vi "State_Machine.vi"(8 "error in (no error)":errorcluster caption="entrée d'erreur (pas d'erreur)", 11 "Generate_SN en entrée":refnum<class "Nodon_Generate_SN_Product.lvclass">) -> (0 "error out":errorcluster caption="sortie d'erreur", 2 "Json_String":string, 3 "Generate_SN en sortie":refnum<class "Nodon_Generate_SN_Product.lvclass">)   [LabVIEW 2020, in "Library Test.lvlib" / "Nodon_Generate_SN_Product.lvclass"]
uses:
  Nodon_Generate_SN_Product.lvclass
  C:/Users/ngarcin/OneDrive - Altyor/Standard TB/Class/Test/Find_SN_In_Database/Find_SN_In_Database.lvclass
  Find_SN_In_Database/Find_SN_In_Database.lvclass
  Nodon_Generate_SN_Product.lvclass/Nodon_Generate_SN_Product.ctl
  Commun VI/Library Commun.lvlib
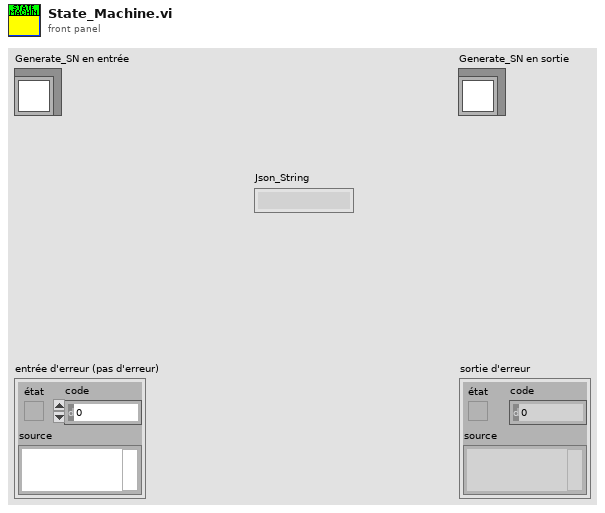
[diagram p1: front panel]
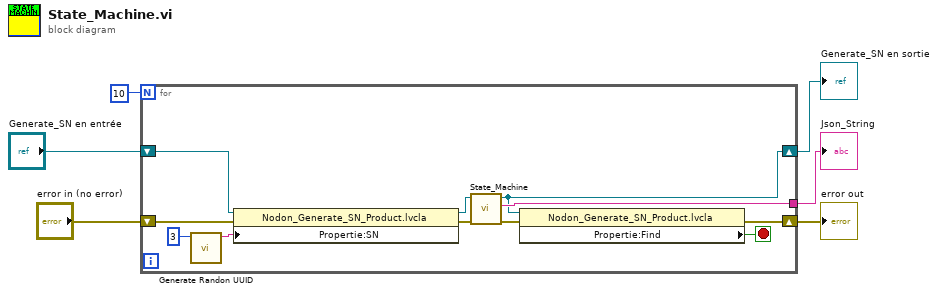
[diagram p0: block diagram]
diagram:
  n1 = for {
    N: 10 -> [_]
    tunnel: [w17] -> w5
    shift-right: [w10] -> w4
    shift-left: "Generate_SN en entrée" -> [w16]
    shift-right: [w9] -> w6
    shift-left: "error in (no error)" -> [w15]
    stop <- w7 stop-if-true
    n2 = call "Generate Randon UUID.vi"("Taille"=3) -> ("chaîne"=w11:string)  [unwired: 10 in]
    n3 = property class="Nodon_Generate_SN_Product.lvcla"(reference=w16, error in=w15, "Propertie:SN"=w11) -> (reference out=w13:refnum<class "Nodon_Generate_SN_Product.lvclass">, error out=w14:errorcluster)
    n4 = call-parent "State_Machine.vi"("error in (no error)"=w14, "Generate_SN en entrée"=w13) -> ("error out"=w8:errorcluster, "Json_String"=w17:string, "Generate_SN en sortie"=w10:refnum<class "Nodon_Generate_SN_Product.lvclass">)  [unwired: 7 in]
    n5 = property class="Nodon_Generate_SN_Product.lvcla"(reference=w10, error in=w8) -> (error out=w9:errorcluster, "Propertie:Find"=w7:bool)  [unwired: 1 out]
  }
  "error out" <- w6
  "Generate_SN en sortie" <- w4
  "Json_String" <- w5
